vi "isNumeric.vi"(8 "error in (no error)":errorcluster, 10 "numberString":string, 11 "DomeCommunicator in":refnum<class "DomeCommunicator.lvclass">) -> (0 "error out":errorcluster, 2 "isNumeric?":bool, 3 "DomeCommunicator out":refnum<class "DomeCommunicator.lvclass">)   [LabVIEW 2016, in "DomeCommunicator.lvclass"]
uses:
  DomeCommunicator.lvclass
  <vilib>/regexp/Match Regular Expression.xnode
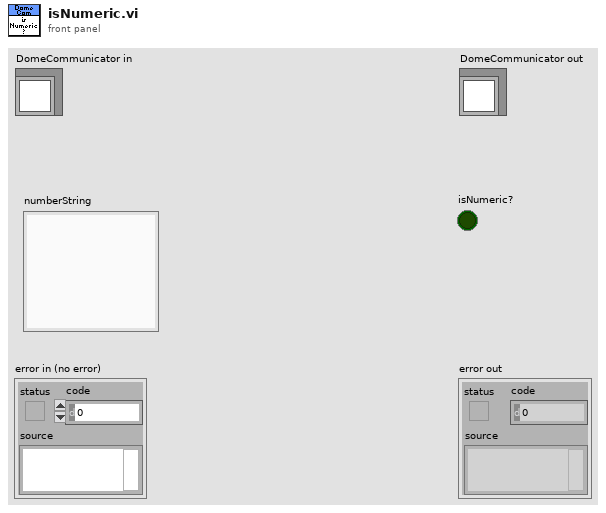
[diagram p1: front panel]
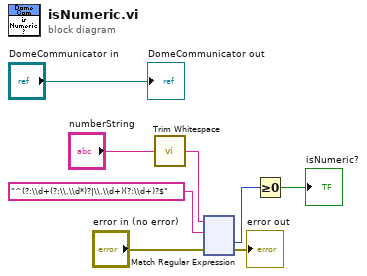
[diagram p0: block diagram]
diagram:
  n1 = call <vilib>:"Trim Whitespace.vi"("string"="numberString") -> ("trimmed string"=w5:string)  [unwired: 1 in]
  n2 = xnode "Match Regular Expression"("input string"=w5, "regular expression"="^(?:\\d+(?:\\.\\d*)?|\\.\\d+)(?:\\d+)?$", "error in"="error in (no error)") -> ("offset past match"=w1:i32, "error out"=→"error out":errorcluster)  [unwired: 3 in, 3 out]
  n3 = Greater Or Equal To 0?(x=w1) -> (x >= 0?=→"isNumeric?":bool)
  "DomeCommunicator out" <- "DomeCommunicator in"
